vi "User Shooter Control.vi"(8 "reinitialize? (F)":bool) -> ()   [LabVIEW 2011]
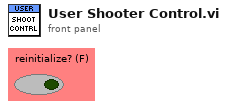
[diagram p1: front panel]
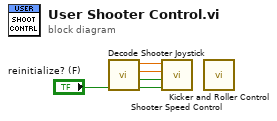
[diagram p0: block diagram]
diagram:
  n1 = call "Decode Shooter Joystick.vi"("reinitialize? (F)"="reinitialize? (F)") -> ("reinitialize"=w4:bool, "full power"=w5:bool, "Bottom RPM"=w1:dbl, "Top RPM"=w2:dbl)  [unwired: 6 in, 1 out]
  n2 = call "Shooter Speed Control.vi"("reinitialize? (F)"=w4, "full power"=w5, "Bottom RPM"=w1, "Top RPM"=w2) -> ()  [unwired: 8 in]
  n3 = call "Kicker and Roller Control.vi"() -> ()  [unwired: 12 in]
